vi "RPC__method Invoke.vi"(8 "error in (no error)":errorcluster, 11 "OOP Server in":refnum<class "Template Server.lvclass">) -> (0 "error out":errorcluster, 3 "OOP Server out":refnum<class "Template Server.lvclass">)   [LabVIEW 2019]
uses:
  Template Server.lvclass
  Template Server.lvclass/Template Server.ctl
  RPC Messages/InvokeResponse/InvokeResponse_Data.ctl
  typeDefs/Server Internal Data.ctl
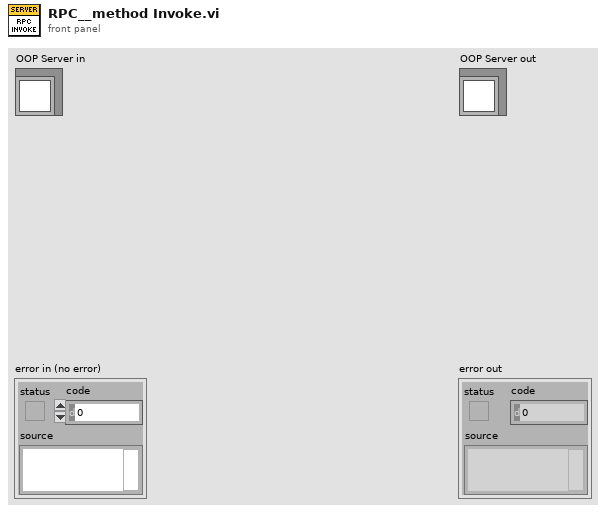
[diagram p1: front panel]
types:
  T1 = typedef "Template Server.lvlib/Template Server.lvclass/InvokeResponse_Data.ctl" = cluster{"Status":i32}
  T2 = typedef "Template Server.lvlib/Template Server.lvclass/Server Internal Data.ctl" = cluster{"Command":string, "Data":variant}
  T3 = typedef "Template Server.lvlib/Template Server.lvclass/Server Internal UEs.ctl" = cluster{"Template Internal UE":refnum<user-event>}
  T4 = typedef "Template Server.lvlib/Template Server.lvclass/Server gRPC UEs.ctl" = cluster{"Template gRPCId UE":T5}
  T5 = typedef "gprc-lvsupport.lvlib/gRPCId Cluster UE.ctl" = refnum<user-event>
  T6 = typedef "gprc-lvsupport.lvlib/grpcId.ctl" = u64
  T7 = typedef "Template Server.lvlib/Template Server.lvclass/InvokeRequest_Data.ctl" = cluster{"command":string, "parameter":string}
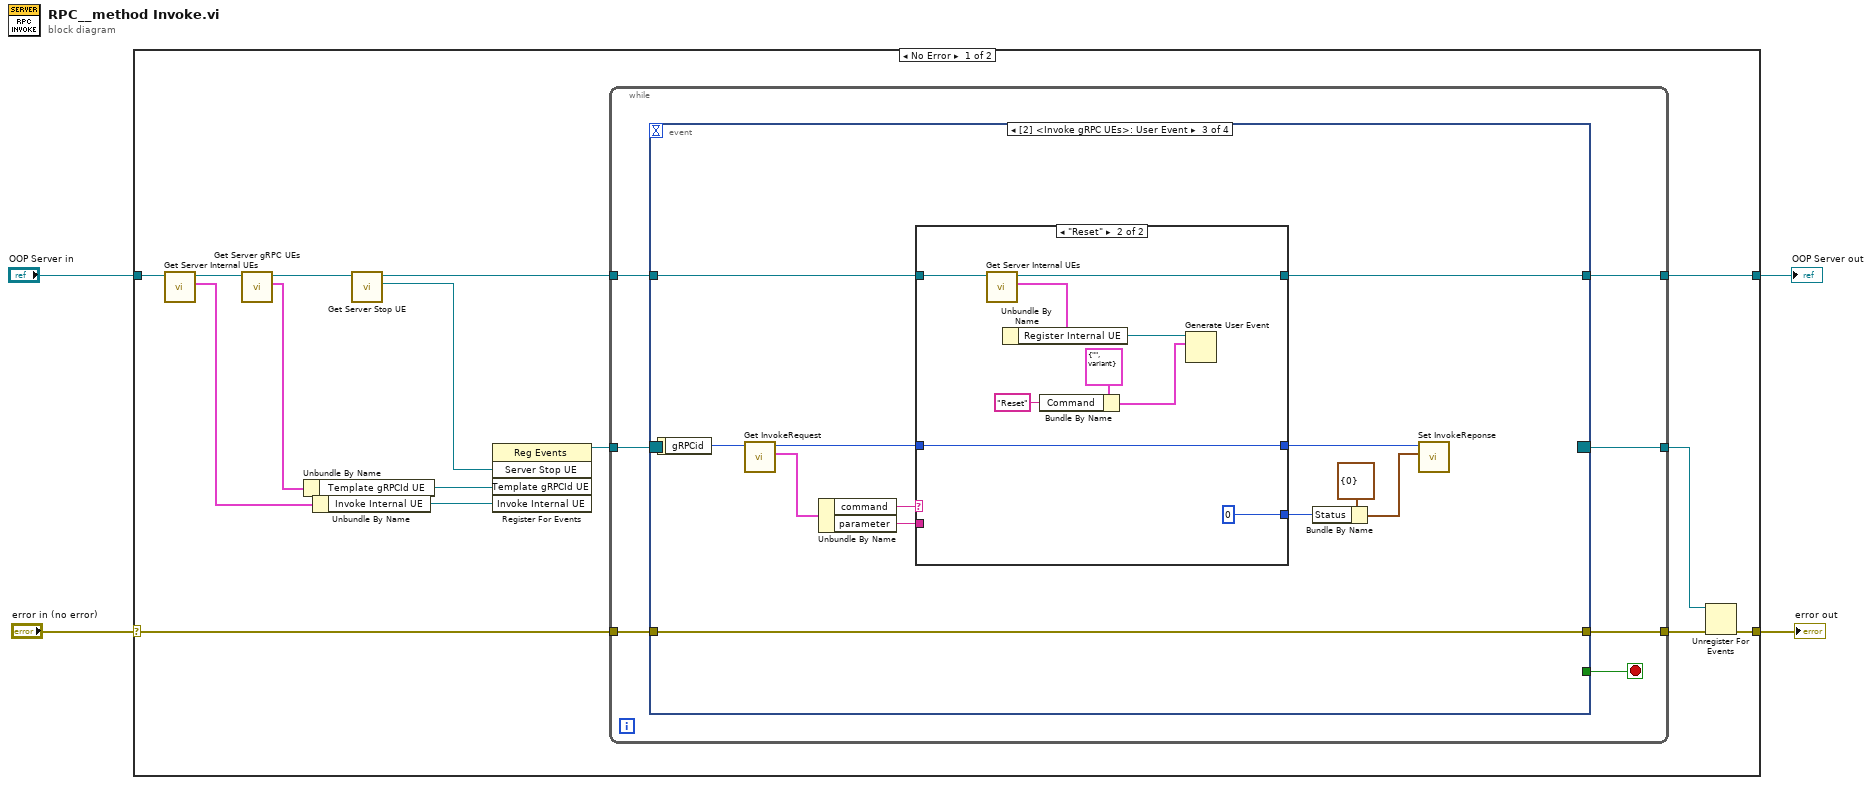
[diagram p0: block diagram]
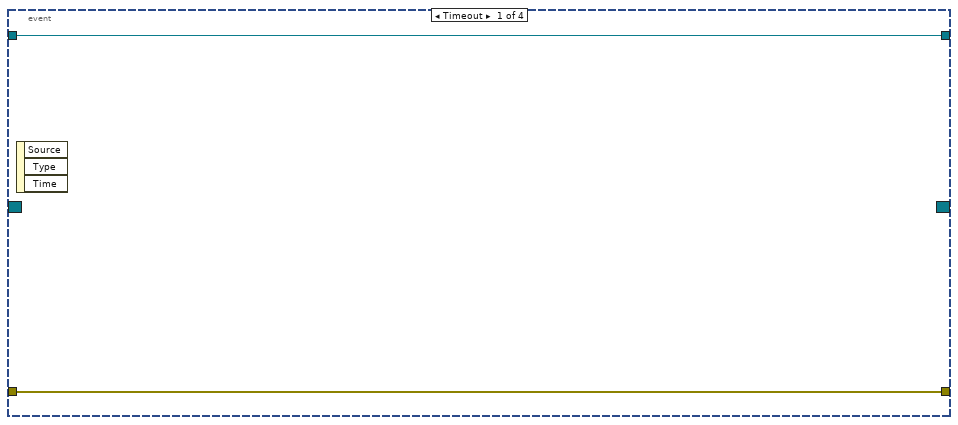
[diagram p2: hidden frame]
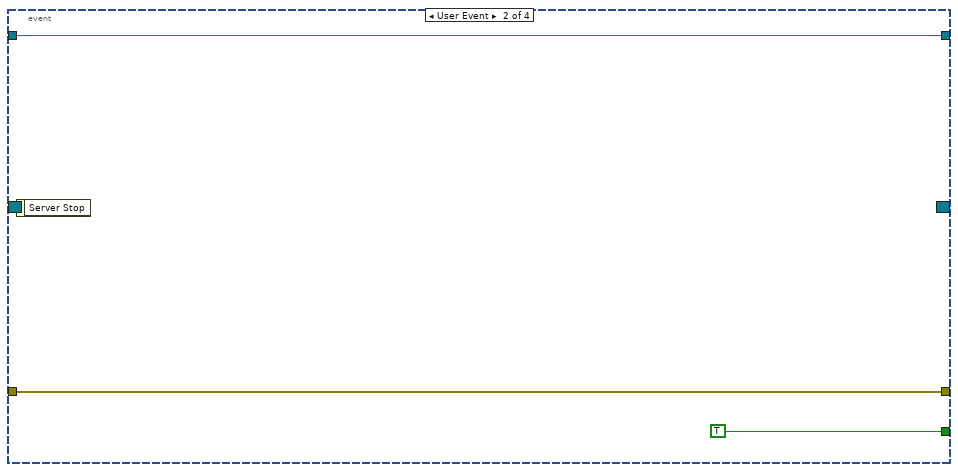
[diagram p3: hidden frame]
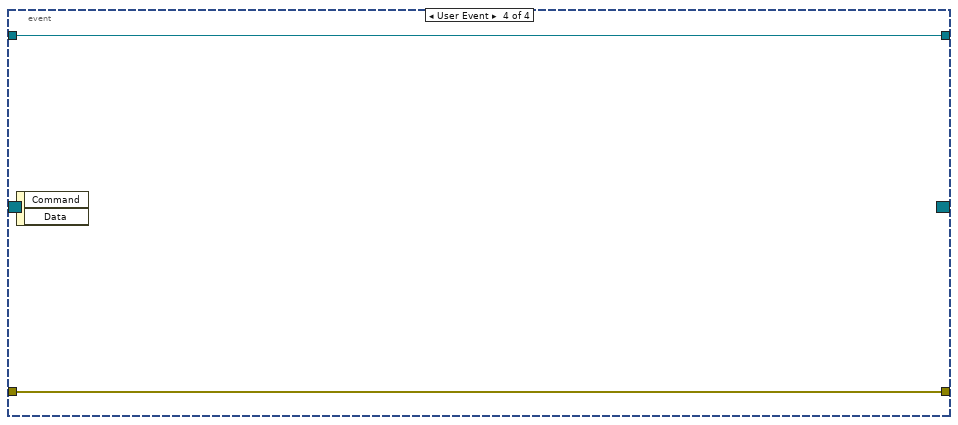
[diagram p5: hidden frame]
diagram:
  n1 = case shown="No Error" "error in (no error)" {
    selector: "error in (no error)" -> [w10 w58]
    tunnel: [w8 w58] -> w3
    tunnel: [w5 w57] -> w1
    tunnel: "OOP Server in" -> [w14 w57]
    frame No Error {
      n2 = call "Get Server Internal UEs.vi"("OOP Server in"=w14) -> ("Server Internal UEs"=w12:T3, "OOP Server out"=w13:refnum<class "Template Server.lvclass">)  [unwired: 9 in]
      n3 = call "Get Server gRPC UEs.vi"("OOP Server in"=w13) -> ("Server gRPC UEs"=w16:T4, "OOP Server out"=w19:refnum<class "Template Server.lvclass">)  [unwired: 9 in]
      n4 = Unbundle By Name(w16) -> ("Template gRPCId UE"=w15:T5)
      n5 = Unbundle By Name(w12) -> ("Invoke Internal UE"=w11:refnum<user-event>)
      n6 = call "Get Server Stop UE.vi"("OOP Server in"=w19) -> ("Server Stop UE"=w18:refnum<user-event>, "OOP Server out"=w6:refnum<class "Template Server.lvclass">)  [unwired: 9 in]
      n7 = register-events(w18, w15, w11) -> (reference out=w17:refnum<event-registration>)  [unwired: 2 in, 1 out]
      n8 = while {
        tunnel: w17 -> [w26]
        tunnel: w10 -> [w24]
        tunnel: [w23] -> w9
        tunnel: [w22] -> w7
        tunnel: w6 -> [w21]
        tunnel: [w20] -> w5
        stop <- w25 stop-if-true
        n9 = event shown="[2] <Invoke gRPC UEs>: User Event" {
          selector: w26 -> [_ _ _ _]
          dyn-events: [_ _ _ _] -> w22
          timeout: _ -> [_ _ _ _]
          tunnel: [_ TRUE _ _] -> w25
          tunnel: w24 -> [w28 w30 w43 w56]
          tunnel: [w28 w30 w43 w56] -> w23
          tunnel: w21 -> [w27 w29 w36 w55]
          tunnel: [w27 w29 w35 w55] -> w20
          event Timeout {
            n10 = event-data() -> ()  [unwired: 1 in, 3 out]
          }
          event User Event {
            n11 = event-data() -> ()  [unwired: 1 in, 1 out]
          }
          event User Event {
            n12 = event-data() -> ("gRPCid"=w42:T6)  [unwired: 1 in]
            n13 = call "Get InvokeRequest.vi"("gRPCid"=w42) -> ("Request Data"=w41:T7, "gRPCid out"=w38:T6)  [unwired: 8 in, 1 out]
            n14 = Unbundle By Name(w41) -> ("command"=w40:string, "parameter"=w39:string)
            n15 = case shown="\"Reset\"" w40 {
              tunnel: w39 -> [_ _]
              tunnel: w38 -> [w45 w52]
              tunnel: [w45 w52] -> w37
              tunnel: w36 -> [w44 w54]
              tunnel: [w44 w53] -> w35
              tunnel: [_ 0 ("Status")] -> w32
              frame "None", Default {
              }
              frame "Reset" {
                n16 = call "Get Server Internal UEs.vi"("OOP Server in"=w54) -> ("Server Internal UEs"=w51:T3, "OOP Server out"=w53:refnum<class "Template Server.lvclass">)  [unwired: 9 in]
                n17 = Unbundle By Name(w51) -> ("Register Internal UE"=w50:refnum<user-event>)
                n18 = Bundle By Name(cluster=T2 {"Command"="", "Data"=variant} ("event data"), "Command"="Reset") -> (w47:T2)
                n19 = Generate User Event(user event=w50, event data cluster=w47) -> ()  [unwired: 2 in, 2 out]
              }
            }
            n20 = Bundle By Name(cluster=T1 {"Status"=0} ("InvokeResponse_Data"), "Status"=w32) -> (w33:T1)
            n21 = call "Set InvokeReponse.vi"("InvokeResponse_Data"=w33, "gRPCid"=w37) -> ()  [unwired: 9 in, 1 out]
          }
          event User Event {
            n22 = event-data() -> ()  [unwired: 1 in, 2 out]
          }
        }
      }
      n23 = Unregister For Events(event registration refnum=w7, error in=w9) -> (error out=w8:errorcluster)
    }
    frame Error {
    }
  }
  "error out" <- w3
  "OOP Server out" <- w1
